vi "Generate Doc.vi"(9 "custom contents options":T1={"include VI connector and icon"=TRUE, "include VI description"=TRUE, "include front panel"=FALSE, "surround front panel with border"=FALSE, "list of controls options"={"include list of controls"=TRUE, "list which controls?"=0, "include control descriptions?"=TRUE, "include control data types?"=TRUE}, "block diagram options"={"include block diagram"=FALSE, "hidden frames"=FALSE, "ordered (repeat from higher level if nested)"=FALSE}, "include VI hierarchy"=FALSE, "include list of subVIs"=FALSE, "include VI history"=FALSE, "include Express VI configuration information"=FALSE} {"list of controls options"."list which controls?" items=["all controls", "connected controls"]}, 10 "Files Generated by Build":path[](array[path]), 11 "appended path":path) -> (0 "error out":errorcluster)   [LabVIEW 2019]
uses:
  <vilib>/printing/EasyPrintingControls.llb/custom_contents_options.ctl
  <vilib>/printing/EasyPrintingControls.llb/list_which_controls.ctl
  <vilib>/Utility/NIReport.llb/Report Type.ctl
  <vilib>/Utility/NIReport.llb/Append Report Text (str wrap).vi
  <vilib>/Utility/NIReport.llb/NI_report.lvclass
  <vilib>/Utility/NIReport.llb/NI_ReportGenerationCore.lvlib
  <vilib>/Ton Plomp/Markdown Report/MarkDownReport.lvclass
panel:
  in  "Examples options":T1={"include VI connector and icon"=FALSE, "include VI description"=TRUE, "include front panel"=TRUE, "surround front panel with border"=TRUE, "list of controls options"={"include list of controls"=FALSE, "list which controls?"=0, "include control descriptions?"=FALSE, "include control data types?"=FALSE}, "block diagram options"={"include block diagram"=TRUE, "hidden frames"=FALSE, "ordered (repeat from higher level if nested)"=FALSE}, "include VI hierarchy"=FALSE, "include list of subVIs"=FALSE, "include VI history"=FALSE, "include Express VI configuration information"=FALSE} {"list of controls options"."list which controls?" items=["all controls", "connected controls"]}
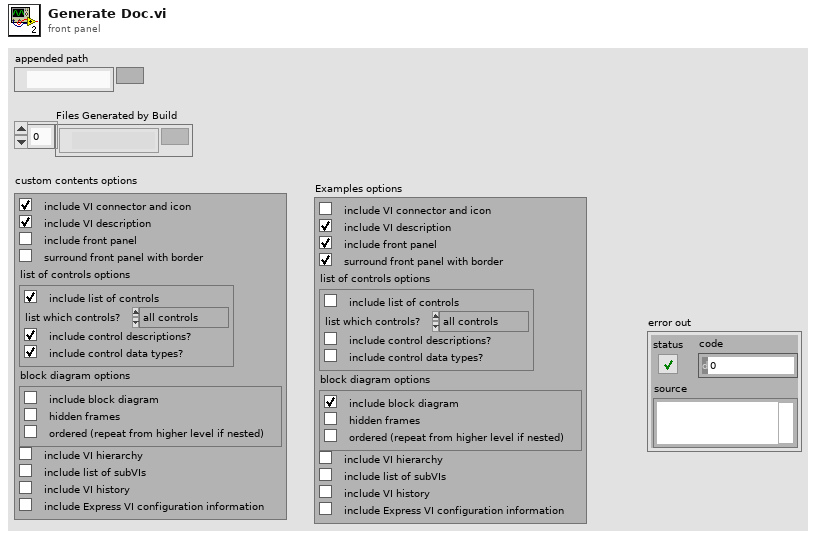
[diagram p1: front panel]
types:
  T1 = typedef "NI_ReportGenerationCore.lvlib/custom_contents_options.ctl" = cluster{"include VI connector and icon":bool, "include VI description":bool, "include front panel":bool, "surround front panel with border":bool, "list of controls options":cluster{"include list of controls":bool, "list which controls?":T2, "include control descriptions?":bool, "include control data types?":bool}, "block diagram options":cluster{"include block diagram":bool, "hidden frames":bool, "ordered (repeat from higher level if nested)":bool}, "include VI hierarchy":bool, "include list of subVIs":bool, "include VI history":bool, "include Express VI configuration information":bool}
  T2 = typedef "NI_ReportGenerationCore.lvlib/list_which_controls.ctl" = u16
  T3 = typedef "NI_ReportGenerationCore.lvlib/Report Type.ctl" = enum16{"HTML", "Word", "Excel"}
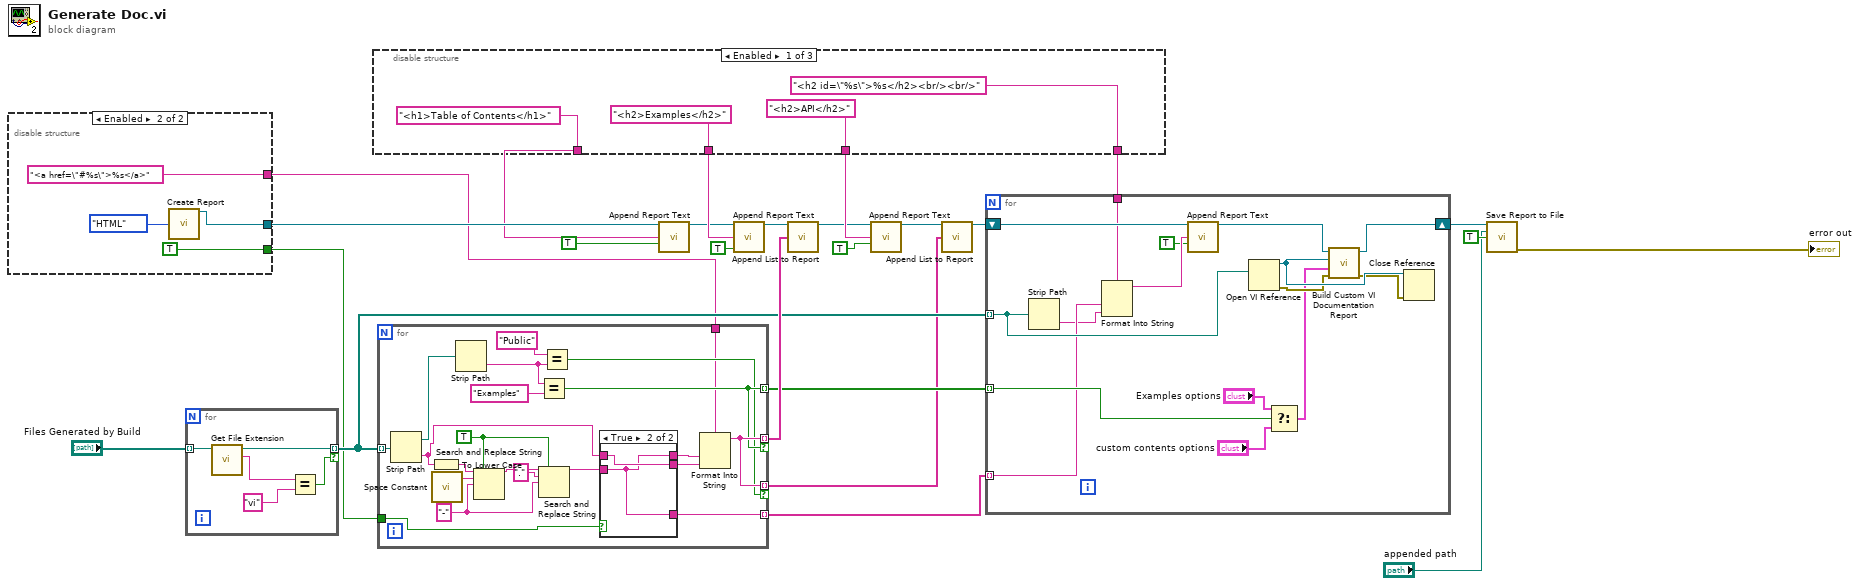
[diagram p0: block diagram]
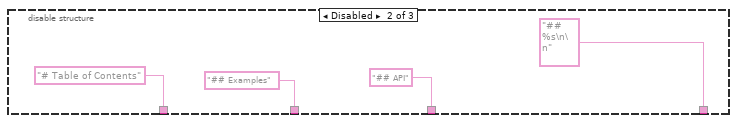
[diagram p2: hidden frame]
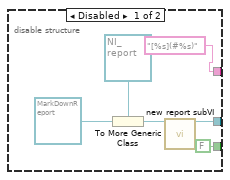
[diagram p5: hidden frame]
diagram:
  n1 = disable-structure shown="Enabled" {
    disable-tunnel: [w28 w35] -> w23
    disable-tunnel: [FALSE TRUE] -> w2
    disable-tunnel: ["[%s](#%s)" ("format string") "<a href=\"#%s\">%s</a>" ("format string")] -> w1
    frame Disabled {
      n2 = To More Generic Class(target class=refnum<class "NI_report.lvclass"> refnum ("NI_report.lvclass"), reference=refnum<class "MarkDownReport.lvclass"> refnum ("Markdown")) -> (generic class reference=w30:refnum<class "NI_report.lvclass">)
      n3 = call-dynamic "new report subVI.vi"("report in"=w30) -> ("report out"=w28:refnum<class "NI_report.lvclass">)  [unwired: 13 in, 1 out]
    }
    frame Enabled {
      n4 = call <vilib>:"Create Report.vi"("report type"=Report_Type."HTML") -> ("report out"=w35:refnum<class "NI_report.lvclass">)  [unwired: 13 in, 1 out]
    }
  }
  n5 = for {
    tunnel: "Files Generated by Build" -> [w40] mode=indexing
    tunnel: [w37] -> w18 mode=indexing if=w36
    n6 = call <vilib>:"Get File Extension.vi"("file"=w40) -> ("lowercase file extension"=w39:string, "dup file"=w37:path)  [unwired: 6 in, 3 out]
    n7 = Equal?(x=w39, y="vi") -> (x = y?=w36:bool)
  }
  n8 = disable-structure shown="Enabled" {
    disable-tunnel: ["<h1>Table of Contents</h1>" ("text") "# Table of Contents" ("text") _] -> w22
    disable-tunnel: ["<h2>Examples</h2>" ("text") "## Examples" ("text") _] -> w13
    disable-tunnel: ["<h2>API</h2>" ("text") "## API" ("text") _] -> w10
    disable-tunnel: ["<h2 id=\"%s\">%s</h2><br/><br/>" ("format string") "## %s\n\n" ("format string") _] -> w4
    frame Enabled {
    }
    frame Disabled {
    }
    frame Disabled {
    }
  }
  n9 = for {
    tunnel: [w58] -> w21 mode=indexing if=w57
    tunnel: w18 -> [w69] mode=indexing
    tunnel: [w57] -> w17 mode=indexing
    tunnel: [w58] -> w15 mode=indexing if=w56
    tunnel: [w49] -> w3 mode=indexing
    tunnel: w2 -> [w54]
    tunnel: w1 -> [w55]
    w64 = TRUE ("Replace All? (false)")
    w65 = "-" ("Replace Pattern (\"\")")
    n10 = Strip Path(path=w69) -> (stripped path=w62:path, name=w52:string)
    n11 = To Lower Case(string=w52) -> (all lower case string=w68:string)
    n12 = call <vilib>:"Space Constant.vi"() -> ("String"=w67:string)
    n13 = Strip Path(path=w62) -> (name=w59:string)  [unwired: 1 out]
    n14 = Search and Replace String(replace all?=w64, input string=w68, search string=w67, replace string=w65) -> (result string=w63:string)  [unwired: 4 in, 3 out]
    n15 = Equal?(x=w59, y="Examples") -> (x = y?=w57:bool)
    n16 = Search and Replace String(replace all?=w64, input string=w63, search string="." ("Search Pattern"), replace string=w65) -> (result string=w53:string)  [unwired: 4 in, 3 out]
    n17 = Equal?(x="Public", y=w59) -> (x = y?=w56:bool)
    n18 = case shown="True" w54 {
      tunnel: w53 -> [w70 w72]
      tunnel: w52 -> [w71 w73]
      tunnel: [w70 w73] -> w51
      tunnel: [w71 w72] -> w50
      tunnel: [_ w72] -> w49
      frame False {
      }
      frame True {
      }
    }
    n19 = Format Into String(format string=w55, w50, w51) -> (resulting string=w58:string)  [unwired: 2 in, 1 out]
  }
  n20 = call-poly <vilib>:"Append Report Text.vi"("report in"=w23, "text"=w22, "append on new line? (F)"=TRUE) -> ("report out"=w12:refnum<class "NI_report.lvclass">)  [unwired: 9 in, 3 out]
  n21 = call-poly <vilib>:"Append Report Text.vi"("report in"=w12, "text"=w13, "append on new line? (F)"=TRUE) -> ("report out"=w11:refnum<class "NI_report.lvclass">)  [unwired: 9 in, 3 out]
  n22 = call-dynamic "Append List to Report.vi"("report in"=w11, "list elements"=w21) -> ("report out"=w8:refnum<class "NI_report.lvclass">)  [unwired: 10 in, 3 out]
  n23 = call-poly <vilib>:"Append Report Text.vi"("report in"=w8, "text"=w10, "append on new line? (F)"=TRUE) -> ("report out"=w7:refnum<class "NI_report.lvclass">)  [unwired: 9 in, 3 out]
  n24 = call-dynamic "Append List to Report.vi"("report in"=w7, "list elements"=w15) -> ("report out"=w16:refnum<class "NI_report.lvclass">)  [unwired: 10 in, 3 out]
  n25 = for {
    shift-right: [w88] -> w24
    shift-left: w16 -> [w85]
    tunnel: w18 -> [w81] mode=indexing
    tunnel: w17 -> [w80] mode=indexing
    tunnel: w4 -> [w76]
    tunnel: w3 -> [w75] mode=indexing
    n26 = Strip Path(path=w81) -> (name=w74:string)  [unwired: 1 out]
    n27 = Format Into String(format string=w76, w75, w74) -> (resulting string=w83:string)  [unwired: 2 in, 1 out]
    n28 = call-poly <vilib>:"Append Report Text.vi"("report in"=w85, "text"=w83, "append on new line? (F)"=TRUE) -> ("report out"=w84:refnum<class "NI_report.lvclass">)  [unwired: 9 in, 3 out]
    n29 = Open VI Reference(vi path=w81) -> (vi reference=w89:refnum<vi>, error out=w86:errorcluster)  [unwired: 5 in]
    n30 = Select(t="Examples options", s=w80, f="custom contents options") -> (s? t:f=w77:T1)
    n31 = call <vilib>:"Build Custom VI Documentation Report.vi"("error in (no error)"=w86, "custom contents options"=w77, "VI reference"=w89, "report in"=w84) -> ("error out"=w87:errorcluster, "report out"=w88:refnum<class "NI_report.lvclass">)  [unwired: 6 out]
    n32 = Close Reference(reference=w89, error in (no error)=w87) -> ()  [unwired: 1 out]
  }
  n33 = call-dynamic "Save Report to File.vi"("report in"=w24, "report file path"="appended path", "prompt to replace? (F)"=TRUE) -> ("error out"=→"error out":errorcluster)  [unwired: 11 in, 1 out]
